vi "startIMU.vi"(0 "MXP Port":enum16{"A", "B"}(ring)) -> (1 "IMU Config Out":T1, 2 "IMU1 SPI Config":T2, 3 "IMU2 SPI Config":T2)   [LabVIEW 2019]
uses:
  SPI/SPI Config.ctl
  IMU Config.ctl
panel:
  in  "IMU Config Reference":T1={"Accelerometer Bias"=[0, 0, 0], "Accelerometer Scale"=0, "Gyro Bias"=[0, 0, 0], "Gyro Scale"=0}
  in  "SPI Config In":T2
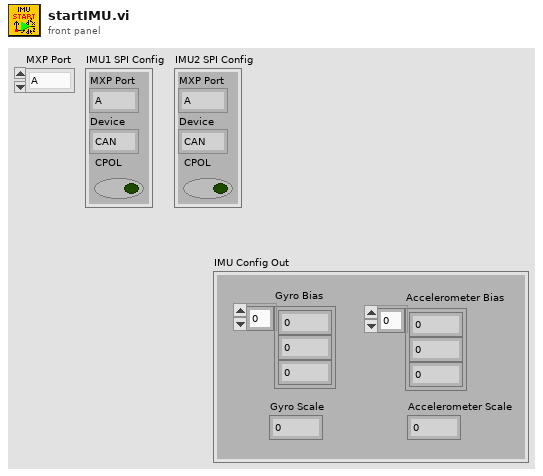
[diagram p1: front panel]
types:
  T1 = typedef "IMU Config.ctl" = cluster{"Accelerometer Bias":i16[], "Accelerometer Scale":i16, "Gyro Bias":i16[], "Gyro Scale":i16}
  T2 = typedef "SPI Config.ctl" = cluster{"MXP Port":enum16{"A", "B"}, "Device":enum16{"CAN", "ENC", "IMU1", "IMU2"}, "CPOL":bool}
  T3 = enum16{"250Hz", "184Hz", "92Hz", "41Hz", "20Hz", "10Hz", "5Hz", "3600Hz"}
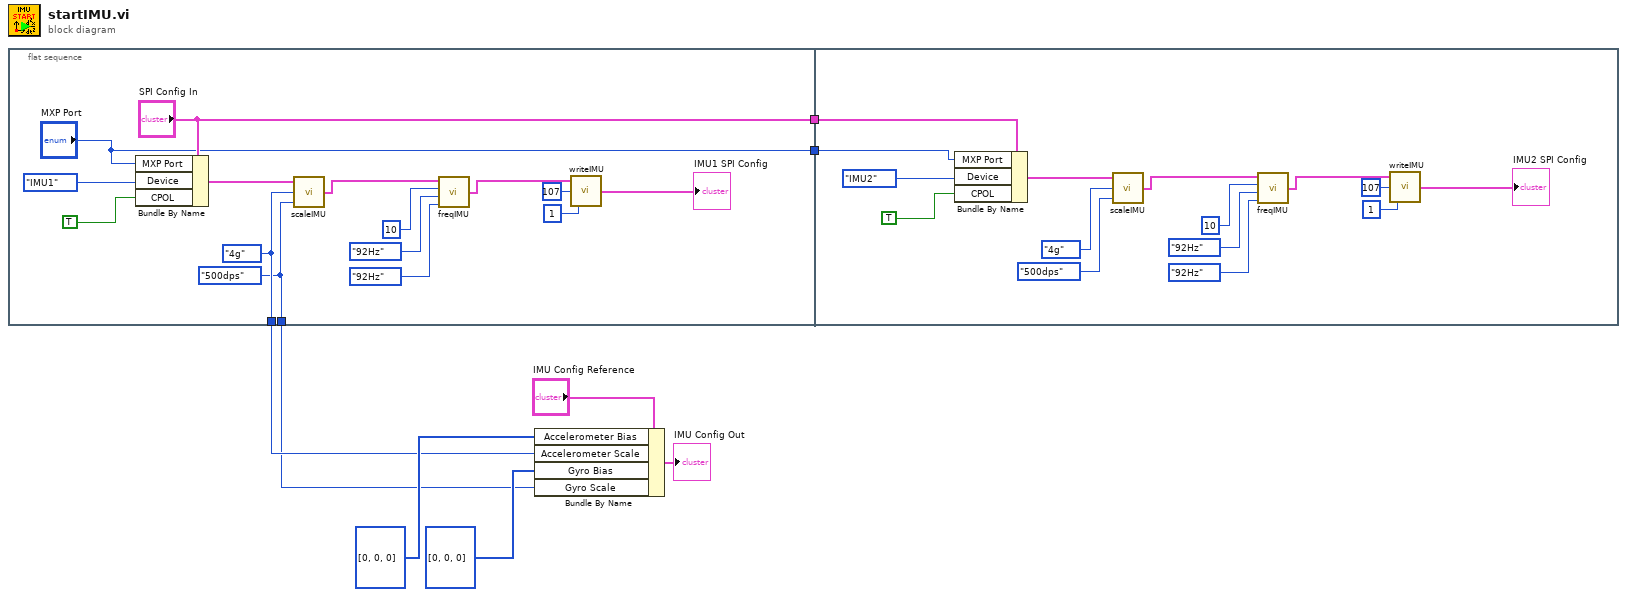
[diagram p0: block diagram]
diagram:
  n1 = flat-sequence {
    tunnel: ["SPI Config In"] -> w8
    tunnel: ["MXP Port"] -> w7
    tunnel: [w10] -> w3
    tunnel: [w9] -> w2
    tunnel: w8 -> [w25]
    tunnel: w7 -> [w24]
    frame #0 {
      w9 = enum16{"250dps", "500dps", "1000dps", "2000dps"}."500dps" ("Gyro Scale")
      w10 = enum16{"2g", "4g", "8g", "16g"}."4g" ("Accel Scale")
      n2 = Bundle By Name(cluster="SPI Config In", "MXP Port"="MXP Port", "Device"=enum16{"CAN", "ENC", "IMU1", "IMU2"}."IMU1", "CPOL"=TRUE) -> (w22:T2)
      n3 = call "scaleIMU.vi"("Gyro Scale"=w9, "Accel Scale"=w10, "SPI Config In"=w22) -> ("SPI Config Out"=w23:T2)
      n4 = call "freqIMU.vi"("Accel DLPF Bandwidth"=T3."92Hz", "Gyro DLPF Bandwidth"=T3."92Hz", "Sample Rate Scaling"=u8 10, "SPI Config In"=w23) -> ("SPI Config Out"=w16:T2)
      n5 = call "writeIMU.vi"("Data"=u8 1, "Address"=u8 107, "SPI Config In"=w16) -> ("SPI Config Out"=→"IMU1 SPI Config":T2)
    }
    frame #1 {
      n6 = Bundle By Name(cluster=w25, "MXP Port"=w24, "Device"=enum16{"CAN", "ENC", "IMU1", "IMU2"}."IMU2", "CPOL"=TRUE) -> (w37:T2)
      n7 = call "scaleIMU.vi"("Gyro Scale"=enum16{"250dps", "500dps", "1000dps", "2000dps"}."500dps", "Accel Scale"=enum16{"2g", "4g", "8g", "16g"}."4g", "SPI Config In"=w37) -> ("SPI Config Out"=w38:T2)
      n8 = call "freqIMU.vi"("Accel DLPF Bandwidth"=T3."92Hz", "Gyro DLPF Bandwidth"=T3."92Hz", "Sample Rate Scaling"=u8 10, "SPI Config In"=w38) -> ("SPI Config Out"=w29:T2)
      n9 = call "writeIMU.vi"("Data"=u8 1, "Address"=u8 107, "SPI Config In"=w29) -> ("SPI Config Out"=→"IMU2 SPI Config":T2)
    }
  }
  n10 = Bundle By Name(cluster="IMU Config Reference", "Accelerometer Bias"=i16[] [0, 0, 0], "Accelerometer Scale"=w3, "Gyro Bias"=i16[] [0, 0, 0] ("Accelerometer Bias"), "Gyro Scale"=w2) -> (→"IMU Config Out":T1)
